vi "FilterWheel.vi"(2 "Filter Wheel":i32(ring)=1 items=["ET520/40"=1, "ET560/50"=2, "ET665Ip"=3, "Quad, 89101m"=4, "empty 1"=5, "empty 2"=6], 3 "FW Serial Port":string(combo)="COM8") -> ()   [LabVIEW 2013]
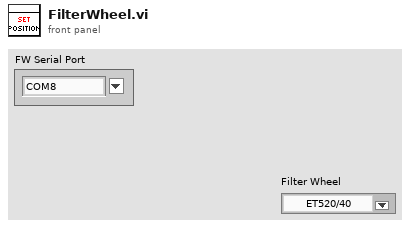
[diagram p1: front panel]
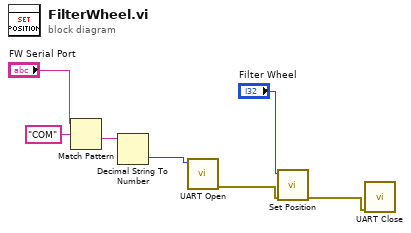
[diagram p0: block diagram]
diagram:
  n1 = Match Pattern(string="FW Serial Port", regular expression="COM") -> (after substring=w6:string)  [unwired: 1 in, 3 out]
  n2 = Decimal String To Number(string=w6) -> (number=w5:i32)  [unwired: 2 in, 1 out]
  n3 = call "UART Open.vi"("Serial Port"=w5) -> ("error out"=w4:errorcluster)  [unwired: 9 in, 1 out]
  n4 = call "Set Position.vi"("error in (no error)"=w4, "Position"="Filter Wheel") -> ("error out"=w3:errorcluster)  [unwired: 9 in]
  n5 = call "UART Close.vi"("error in (no error)"=w3) -> ()  [unwired: 10 in, 1 out]
